vi "Remove Line.vi"(8 "error in (no error)":errorcluster, 10 "Active Line Name":string, 11 "object Refs in":T1) -> (0 "error out":errorcluster, 3 "object Refs out":T1)   [LabVIEW 2014, in "Modbus Module editor node.lvclass"]
uses:
  Modbus Module editor node.lvclass
  <vilib>/NI/DCAF/Tag Editor Core/Table API/Table Manager/object ref.ctl
  <vilib>/NI/DCAF/Tag Editor Core/Configuration Editor/Classes/Engine Parent/Engine Parent Editor Node.lvclass
  <vilib>/NI/DCAF/Tag Editor Core/Configuration Editor/Classes/Module editor node/module editor node.lvclass
  module/configuration/Modbus Module configuration.lvclass
  module/module channel/Modbus Module Channel.lvclass
  <vilib>/NI/Configuration Framework/serializable configuration/NISE_CEF_serializable configuration.lvclass/NISE_CEF_serializable configuration.ctl
  <vilib>/Utility/LVClass/Get LV Class Name.vi
  <vilib>/NI/Configuration Framework/error generator/NISE_error generator.vi
  <vilib>/NI/Module Execution Interface/Engine Configuration/engine configuration.lvclass
  <vilib>/NI/Configuration Framework/serializable configuration/NISE_CEF_serializable configuration.lvclass
  <vilib>/NI/DCAF/Tag Editor Core/Table API/Table Manager/Table Manager.lvclass
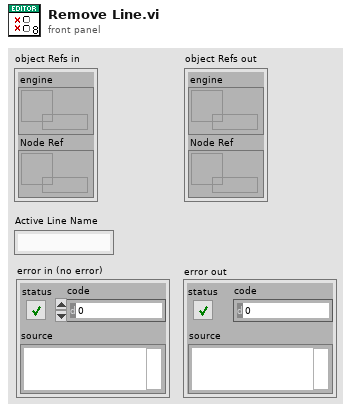
[diagram p1: front panel]
types:
  T1 = typedef "Table Manager.lvlib/Table Manager.lvclass/object ref.ctl" = cluster{"engine":refnum<data-value>, "Node Ref":refnum<data-value>}
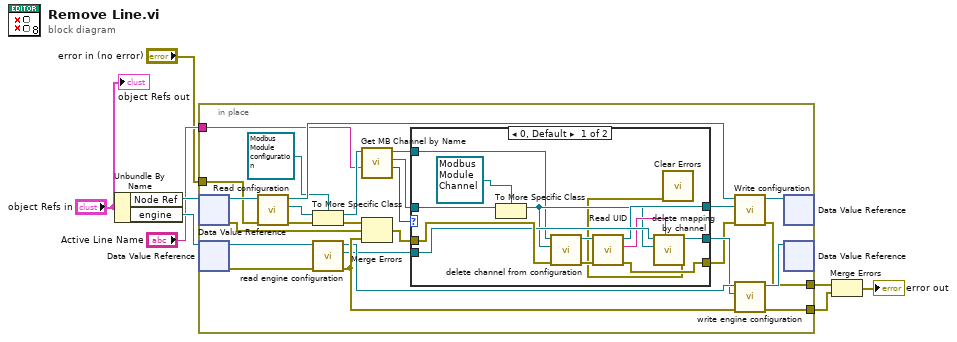
[diagram p0: block diagram]
diagram:
  n1 = Unbundle By Name("object Refs in") -> ("Node Ref"=w4:refnum<data-value>, "engine"=w5:refnum<data-value>)
  n2 = in-place {
    in-place-border: [w29] -> w7
    in-place-border: "Active Line Name" -> [w12]
    in-place-border: "error in (no error)" -> [w17]
    in-place-border: [w13] -> w1
    n3 = in-place-dvr #1(w4) -> (w21:refnum<class "module editor node.lvclass">, w28:errorcluster)
    n4 = in-place-dvr #2(w5) -> (w34:refnum<class "Engine Parent Editor Node.lvclass">, w33:errorcluster)
    n5 = call-dynamic "Read configuration.vi"("error in"=w17, "NISE_CEF_serializable node in"=w21) -> ("error out"=w16:errorcluster, "configuration"=w25:refnum<class "NISE_CEF_serializable configuration.lvclass">, "NISE_CEF_serializable node out"=w22:refnum<class "module editor node.lvclass">)  [unwired: 7 in]
    n6 = To More Specific Class(target class=refnum<class "Modbus Module configuration.lvclass"> refnum ("Modbus Slave configuration in"), reference=w25, error in=w16) -> (specific class reference=w19:refnum<class "Modbus Module configuration.lvclass">, error out=w15:errorcluster)
    n7 = call <vilib>:"read engine configuration.vi"("error in"=w33, "Engine Parent Editor Node in"=w34) -> ("error out"=w31:errorcluster, "engine configuration"=w18:refnum<class "engine configuration.lvclass">, "Engine Parent Editor Node out"=w30:refnum<class "Engine Parent Editor Node.lvclass">)  [unwired: 7 in]
    n8 = call "Get MB Channel by Name.vi"("Active Line Name"=w12, "Modbus Module configuration in"=w19) -> ("index"=w11:i32, "Modbus Module Channel.lvclass"=w9:refnum<class "Modbus Module Channel.lvclass">, "Modbus Module configuration out"=w10:refnum<class "Modbus Module configuration.lvclass">)  [unwired: 6 in, 1 out]
    n9 = Merge Errors(w15, w28, w31) -> (w27:errorcluster)
    n10 = case shown="0, Default" w11 {
      tunnel: [w36 w49] -> w14
      tunnel: w18 -> [w44 w50]
      tunnel: w27 -> [w47 w49]
      tunnel: [w43 w50] -> w26
      tunnel: [w42 w48] -> w23
      tunnel: w10 -> [w37 w48]
      tunnel: w9 -> [w40 _]
      frame 0, Default {
        n11 = To More Specific Class(target class=refnum<class "Modbus Module Channel.lvclass"> refnum ("Modbus Module Channel.lvclass"), reference=w40) -> (specific class reference=w38:refnum<class "Modbus Module Channel.lvclass">)  [unwired: 1 in, 1 out]
        n12 = call "delete channel from configuration.vi"("error in"=w47, "Modbus Module Channel.lvclass"=w38, "Modbus Slave configuration in"=w37) -> ("error out"=w45:errorcluster, "Modbus Slave configuration out"=w46:refnum<class "Modbus Module configuration.lvclass">)  [unwired: 7 in]
        n13 = call <vilib>:"Read UID.vi"("error in"=w45, "configuration in"=w46) -> ("error out"=w36:errorcluster, "instance id"=w39:string, "configuration out"=w42:refnum<class "Modbus Module configuration.lvclass">)  [unwired: 7 in]
        n14 = call <vilib>:"delete mapping by channel.vi"("owner ID"=w39, "channel"=w38, "engine configuration in"=w44) -> ("error out"=w35:errorcluster, "engine configuration out"=w43:refnum<class "engine configuration.lvclass">)  [unwired: 7 in]
        n15 = call <vilib>:"Clear Errors.vi"("error in (no error)"=w35) -> ()  [unwired: 5 in, 2 out]
      }
      frame 1 {
      }
    }
    n16 = call-dynamic "Write configuration.vi"("error in"=w14, "configuration"=w23, "NISE_CEF_serializable node in"=w22) -> ("error out"=w13:errorcluster, "NISE_CEF_serializable node out"=w24:refnum<class "module editor node.lvclass">)  [unwired: 7 in]
    n17 = call <vilib>:"write engine configuration.vi"("error in"=w31, "engine configuration"=w26, "Engine Parent Editor Node in"=w30) -> ("error out"=w29:errorcluster, "Engine Parent Editor Node out"=w32:refnum<class "Engine Parent Editor Node.lvclass">)  [unwired: 7 in]
    n18 = in-place-dvr #1(w24) -> ()  [unwired: 2 out]
    n19 = in-place-dvr #2(w32) -> ()  [unwired: 2 out]
  }
  n20 = Merge Errors(w1, w7) -> (→"error out":errorcluster)
  "object Refs out" <- "object Refs in"
